vi "GetWrapped.vi"(11 "Input":string) -> (1 "offset after":i32, 3 "Expression":string)   [LabVIEW 2012]
uses:
  <vilib>/regexp/Match Regular Expression.xnode
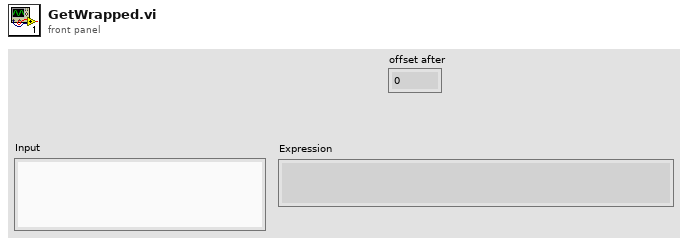
[diagram p1: front panel]
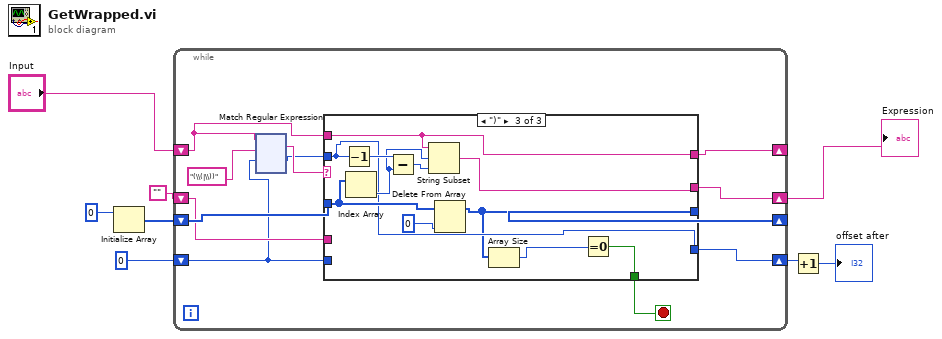
[diagram p0: block diagram]
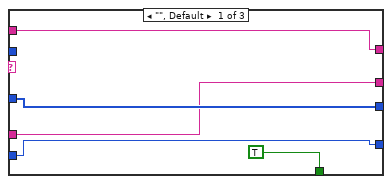
[diagram p2: hidden frame]
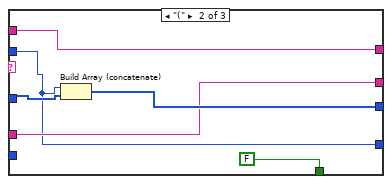
[diagram p3: hidden frame]
diagram:
  n1 = Initialize Array(0) -> (w2:i32[])  [unwired: 1 in]
  n2 = while {
    shift-right: [w20] -> _
    shift-left: w2 -> [w13]
    shift-right: [w19] -> _
    shift-left: "Input" -> [w17]
    shift-right: [w12] -> w7
    shift-left: "" -> [w11]
    shift-right: [w10] -> w6
    shift-left: 0 -> [w9]
    stop <- w18 stop-if-true
    n3 = xnode "Match Regular Expression"("input string"=w17, "regular expression"="(\\(|\\))", "offset (0)"=w9) -> ("whole match"=w15:string, "offset past match"=w14:i32)  [unwired: 3 in, 3 out]
    n4 = case shown="\")\"" w15 {
      tunnel: w13 -> [w136 w139 w153]
      tunnel: [w136 w142 w145] -> w20
      tunnel: w14 -> [_ w137 w146]
      tunnel: w17 -> [w134 w140 w148]
      tunnel: [w134 w140 w148] -> w19
      tunnel: [TRUE FALSE w144] -> w18
      tunnel: [w133 w138 w147] -> w12
      tunnel: w11 -> [w133 w138 _]
      tunnel: w9 -> [w132 _ _]
      tunnel: [w132 w137 w146] -> w10
      frame "", Default {
      }
      frame "(" {
        n5 = Build Array (concatenate)(w137, w139) -> (w142:i32[])
      }
      frame ")" {
        n6 = Decrement(x=w146) -> (x-1=w151:i32)
        n7 = Index Array(array=w153) -> (element=w150:i32)  [unwired: 1 in]
        n8 = Subtract(x=w151, y=w150) -> (x-y=w152:i32)
        n9 = String Subset(string=w148, offset (0)=w150, length (rest)=w152) -> (substring=w147:string)
        n10 = Delete From Array(array=w153, index=0) -> (array with subset deleted=w145:i32[])  [unwired: 1 in, 1 out]
        n11 = Array Size(array=w145) -> (size(s)=w143:i32)
        n12 = Equal To 0?(x=w143) -> (x = 0?=w144:bool)
      }
    }
  }
  "Expression" <- w7
  n13 = Increment(x=w6) -> (x+1=→"offset after":i32)
